vi "Get Wheel Parameter by Name as String.vi"(8 "error in (no error)":errorcluster, 10 "parameter name":string, 11 "wheel in":refnum<class "NI_Robotics_Steering Wheel.lvclass">) -> (0 "error out":errorcluster, 1 "found?":bool, 2 "parameter value":string, 3 "wheel out":refnum<class "NI_Robotics_Steering Wheel.lvclass">)   [LabVIEW 2017, in "NI_Robotics_Steering Wheel.lvclass"]
uses:
  <vilib>/robotics/Steering/Steering Wheel/NI_Robotics_Steering Wheel.lvclass
  <vilib>/robotics/Steering/Steering Wheel/NI_Robotics_Steering Wheel.lvclass/NI_Robotics_Steering Wheel.ctl
  <vilib>/robotics/Actuation/Motor Communication/NI_Robotics_Motor Communication.lvclass/NI_Robotics_Motor Communication.ctl
  <vilib>/robotics/Steering/Wheel/NI_Robotics_Wheel.lvclass
  <vilib>/robotics/Actuation/Motor Communication/NI_Robotics_Motor Communication.lvclass
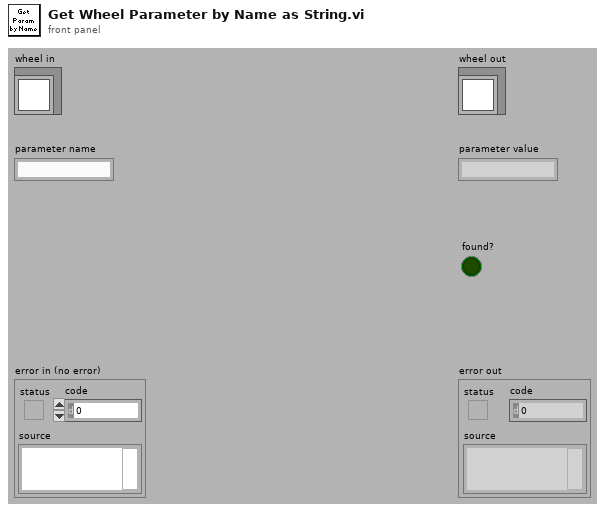
[diagram p1: front panel]
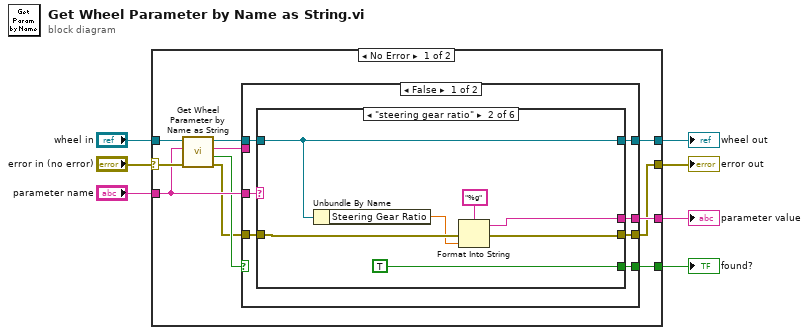
[diagram p0: block diagram]
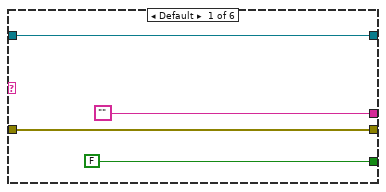
[diagram p2: hidden frame]
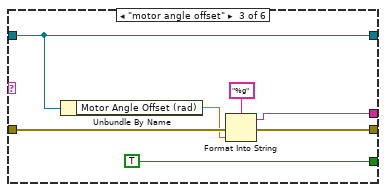
[diagram p3: hidden frame]
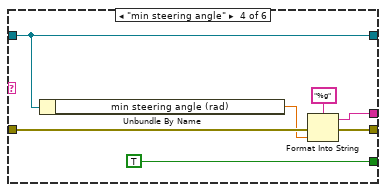
[diagram p4: hidden frame]
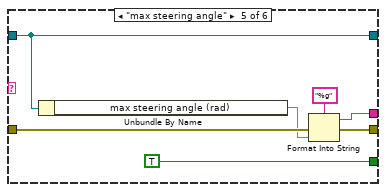
[diagram p5: hidden frame]
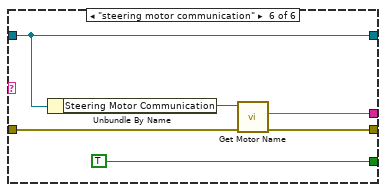
[diagram p6: hidden frame]
diagram:
  n1 = case shown="No Error" "error in (no error)" {
    selector: "error in (no error)" -> [w17 w68]
    tunnel: [w8 w68] -> w4
    tunnel: [w10 _] -> w1
    tunnel: [w13 _] -> w2
    tunnel: [w14 w69] -> w3
    tunnel: "parameter name" -> [w12 _]
    tunnel: "wheel in" -> [w18 w69]
    frame No Error {
      n2 = call-parent "Get Wheel Parameter by Name as String.vi"("error in (no error)"=w17, "parameter name"=w12, "wheel in"=w18) -> ("error out"=w9:errorcluster, "found?"=w11:bool, "parameter value"=w16:string, "wheel out"=w15:refnum<class "NI_Robotics_Steering Wheel.lvclass">)  [unwired: 5 in]
      n3 = case shown="False" w11 {
        selector: w11 -> [_ w65]
        tunnel: w16 -> [_ w66]
        tunnel: w15 -> [w25 w67]
        tunnel: [w23 w67] -> w14
        tunnel: [w22 w66] -> w13
        tunnel: w12 -> [w24 _]
        tunnel: [w21 w65] -> w10
        tunnel: w9 -> [w20 w64]
        tunnel: [w19 w64] -> w8
        frame False {
          n4 = case shown="\"steering gear ratio\"" w24 {
            tunnel: w25 -> [w29 w36 w43 w50 w57 w63]
            tunnel: [w29 w36 w43 w50 w57 w63] -> w23
            tunnel: ["" ("parameter value") w32 w37 w44 w51 w58] -> w22
            tunnel: [FALSE TRUE TRUE TRUE TRUE TRUE] -> w21
            tunnel: w20 -> [w26 w34 w40 w47 w54 w60]
            tunnel: [w26 w33 w39 w46 w53 w59] -> w19
            frame Default {
            }
            frame "steering gear ratio" {
              n5 = Unbundle By Name(w36) -> ("Steering Gear Ratio"=w31:dbl)
              n6 = Format Into String(format string="%g", error in=w34, w31) -> (resulting string=w32:string, error out=w33:errorcluster)  [unwired: 1 in]
            }
            frame "motor angle offset" {
              n7 = Unbundle By Name(w43) -> ("Motor Angle Offset (rad)"=w38:dbl)
              n8 = Format Into String(format string="%g", error in=w40, w38) -> (resulting string=w37:string, error out=w39:errorcluster)  [unwired: 1 in]
            }
            frame "min steering angle" {
              n9 = Unbundle By Name(w50) -> ("min steering angle (rad)"=w45:dbl)
              n10 = Format Into String(format string="%g", error in=w47, w45) -> (resulting string=w44:string, error out=w46:errorcluster)  [unwired: 1 in]
            }
            frame "max steering angle" {
              n11 = Unbundle By Name(w57) -> ("max steering angle (rad)"=w52:dbl)
              n12 = Format Into String(format string="%g", error in=w54, w52) -> (resulting string=w51:string, error out=w53:errorcluster)  [unwired: 1 in]
            }
            frame "steering motor communication" {
              n13 = Unbundle By Name(w63) -> ("Steering Motor Communication"=w61:refnum<class "NI_Robotics_Motor Communication.lvclass">)
              n14 = call <vilib>:"Get Motor Name.vi"("error in (no error)"=w60, "motor communication in"=w61) -> ("error out"=w59:errorcluster, "motor name"=w58:string)  [unwired: 7 in, 1 out]
            }
          }
        }
        frame True {
        }
      }
    }
    frame Error {
    }
  }
  "error out" <- w4
  "wheel out" <- w3
  "found?" <- w1
  "parameter value" <- w2
